vi "Execute Command.vi"(8 "error in (no error)":errorcluster, 10 "command":T1, 11 "Dispatcher in":refnum<class "Dispatcher Thread.lvclass">) -> (0 "error out":errorcluster, 3 "Dispatcher out":refnum<class "Dispatcher Thread.lvclass">)   [LabVIEW 2017, in "DSF Core.lvlib" / "Dispatcher Thread.lvclass"]
uses:
  Dispatcher Thread.lvclass
  Interfaces/Dispatcher/Command Data.ctl
  Interfaces/Dispatcher/Command.ctl
  Interfaces/Dispatcher/Parameters.ctl
  Interfaces/Dispatcher/Dispatcher Interface.lvclass
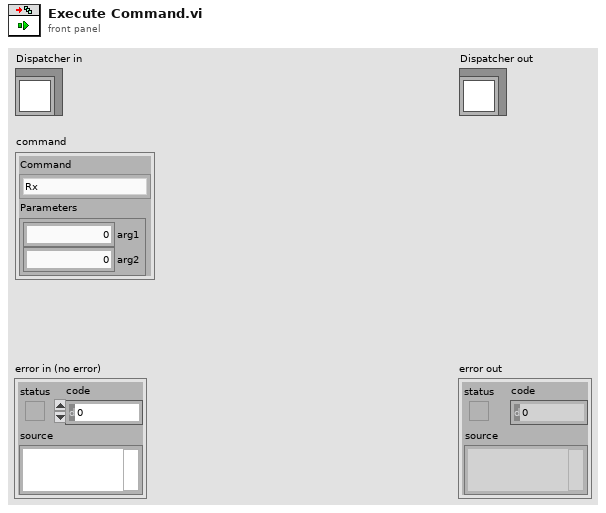
[diagram p1: front panel]
types:
  T1 = typedef "DSF Core.lvlib/Dispatcher Interface.lvclass/Command Data.ctl" = cluster{"Command":T2, "Parameters":T3}
  T2 = typedef "DSF Core.lvlib/Dispatcher Interface.lvclass/Command.ctl" = enum8{"Rx", "Tx", "Set Inline Buffer", "Shutdown"}
  T3 = typedef "DSF Core.lvlib/Dispatcher Interface.lvclass/Parameters.ctl" = cluster{"arg1":u64, "arg2":u64}
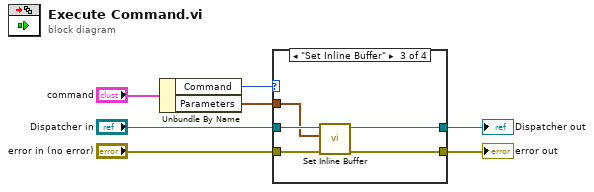
[diagram p0: block diagram]
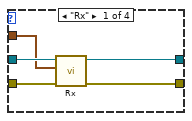
[diagram p2: hidden frame]
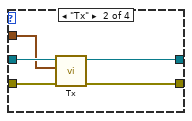
[diagram p3: hidden frame]
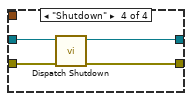
[diagram p4: hidden frame]
diagram:
  n1 = Unbundle By Name("command") -> ("Command"=w2:T2, "Parameters"=w1:T3)
  n2 = case shown="\"Set Inline Buffer\"" w2 {
    tunnel: "Dispatcher in" -> [w12 w17 w19 w26]
    tunnel: [w10 w15 w22 w24] -> w6
    tunnel: "error in (no error)" -> [w11 w16 w20 w25]
    tunnel: [w9 w14 w21 w23] -> w5
    tunnel: w1 -> [w8 w13 w18 _]
    frame "Rx" {
      n3 = call "Rx.vi"("error in (no error)"=w11, "Command Parameters"=w8, "Dispatcher in"=w12) -> ("error out"=w9:errorcluster, "Dispatcher out"=w10:refnum<class "Dispatcher Thread.lvclass">)  [unwired: 7 in]
    }
    frame "Tx" {
      n4 = call "Tx.vi"("error in (no error)"=w16, "Command Parameters"=w13, "Dispatcher in"=w17) -> ("error out"=w14:errorcluster, "Dispatcher out"=w15:refnum<class "Dispatcher Thread.lvclass">)  [unwired: 7 in]
    }
    frame "Set Inline Buffer" {
      n5 = call "Set Inline Buffer.vi"("error in (no error)"=w20, "Command Parameters"=w18, "Dispatcher in"=w19) -> ("error out"=w21:errorcluster, "Dispatcher out"=w22:refnum<class "Dispatcher Thread.lvclass">)  [unwired: 7 in]
    }
    frame "Shutdown" {
      n6 = call "Dispatch Shutdown.vi"("error in (no error)"=w25, "Dispatcher in"=w26) -> ("error out"=w23:errorcluster, "Dispatcher out"=w24:refnum<class "Dispatcher Thread.lvclass">)  [unwired: 8 in]
    }
  }
  "error out" <- w5
  "Dispatcher out" <- w6
